vi "StahlPS_Pbus.constructor.vi"(0 "name":string, 2 "data in":string, 5 "error in(no error)":errorcluster) -> (14 "i ref out":refnum<vi>, 16 "data out":string, 19 "error out":errorcluster)   [LabVIEW 2014, in "StahlPS_Pbus.lvlib"]
doc: "This is the constructor of a class.\n\nLicense Agreement for this software:\n\nCopyright (C)\nGesellschaft für Schwerionenforschung, GSI\nPlanckstr. 1\n64291 Darmstadt\nGermany\n\nContact: D.Beck@gsi.de \n\nThis program is free software; you can redistribute it and/or modify it under the terms of the \nGNU General Public License as published by the Free Software Foundation; either version 2 of \nthe license, or (at your option) any later version.\n\nThis program is distributed in the hope that it will be useful, but WITHOUT ANY WARRANTY; \nwithout even the implied warranty of MERCHANTABILITY or FITNESS FOR A PARTICULAR PURPOSE. See the GNU General License for more details (http://www.gnu.org).\n\nGesellschaft für Schwerionenforschung, GSI\nPlanckstr. 1, 64291 Darmstadt, Germany\nFor all questions and ideas contact: M.Richter@gsi.de, H.Brand@gsi.de or D.Beck@gsi.de.\nLast update: 16-JUN-2004"
uses:
  StahlPS_Pbus.lvlib
  CSCore/CSApplicationBaseClasses/DeviceBase/DeviceBase.myEventNames.ctl
  CSCore/CSApplicationBaseClasses/PSChannelBase/PSChannelBase.myEventNames.ctl
  CSlibraries/UtilityLib/UtilityLib.valueStatus.ctl
  CSCore/CSSystem/CSSystemLib/CSSystemLib.lvlib
  CSCore/CSApplicationBaseClasses/PSChannelBase/PSChannelBase.lvlib
  CSCore/CSApplicationBaseClasses/DeviceBase/DeviceBase.lvlib
  CSlibraries/UtilityLib/UtilityLib.lvlib
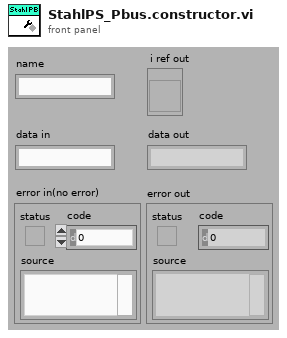
[diagram p1: front panel]
types:
  T1 = typedef "UtilityLib.lvlib/UtilityLib.valueStatus.ctl" = enum16{"no info available", "stand by/off", "on", "warning", "alarm/malfunction", "not implemented", "user action required", "important information", "system default", "control default", "indicator default", "button default"}
  T2 = enum16{"SetAttribute", "GetAttribute", "CreateAttribute", "DestroyAttribute", "DestroyAllAtributes"}
  T3 = typedef "PSChannelBase.lvlib/PSChannelBase.myEventNames.ctl" = enum16{"lvmsg://EmergencyOff", "lvmsg://SetOnOff", "lvmsg://GetOnOff", "lvmsg://SetVoltage", "lvmsg://GetVoltage", "lvmsg://SetCurrent", "lvmsg://GetCurrent", "lvmsg://SetTripCurrent", "lvmsg://GetTripCurrent", "lvmsg://SetRampUpSpeed", "lvmsg://GetRampUpSpeed", "lvmsg://SetRampDownSpeed", "lvmsg://GetRampDownSpeed", "lvmsg://SetChannelOnOff", "lvmsg://GetChannelOnOff", "lvmsg://SetChannelVoltage", "lvmsg://GetChannelVoltage", "lvmsg://SetChannelCurrent", "lvmsg://GetChannelCurrent", "lvmsg://SetChannelTripCurrent", "lvmsg://GetChannelTripCurrent", "lvmsg://SetChannelRampUpSpeed", "lvmsg://GetChannelRampUpSpeed", "lvmsg://SetChannelRampDownSpeed", "lvmsg://GetChannelRampDownSpeed"}
  T4 = typedef "DeviceBase.lvlib/DeviceBase.myEventNames.ctl" = enum16{"lvmsg://Initialize", "lvmsg://Close", "lvmsg://Configure", "lvmsg://Reset", "lvmsg://IDQuery"}
  T5 = typedef "StahlPS_Pbus.lvlib/StahlPS_Pbus.i attribute.ctl" = cluster{"Type":string, "CALC_FACTOR_SET_VOLTAGE":dbl, "CALC_FACTOR_GET_VOLTAGE":dbl, "CALC_FACTOR_GET_CURRENT":dbl, "CALC_FACTOR_SET_CURRENT ":dbl, "REG_VALUE":dbl, "Sign":bool, "setVoltIDs":i32[], "Elektrode Names":string[]}
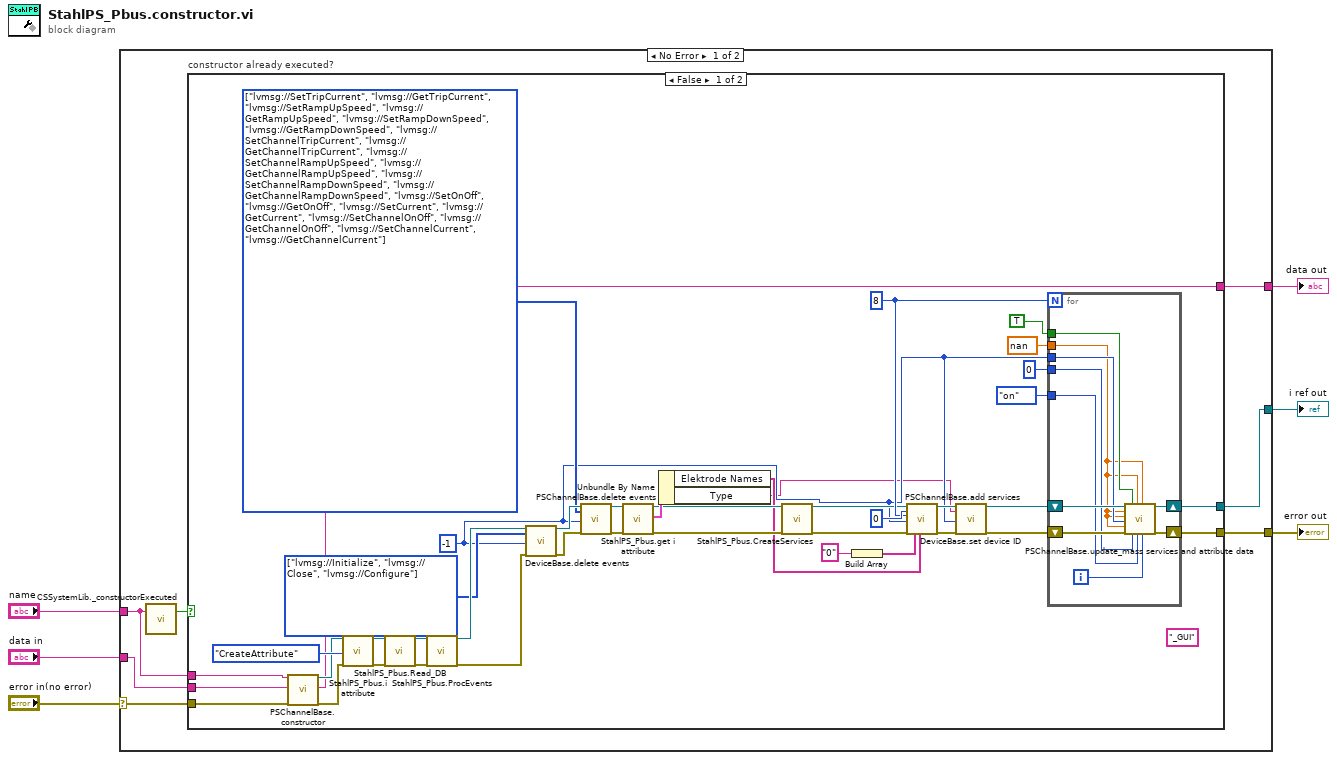
[diagram p0: block diagram]
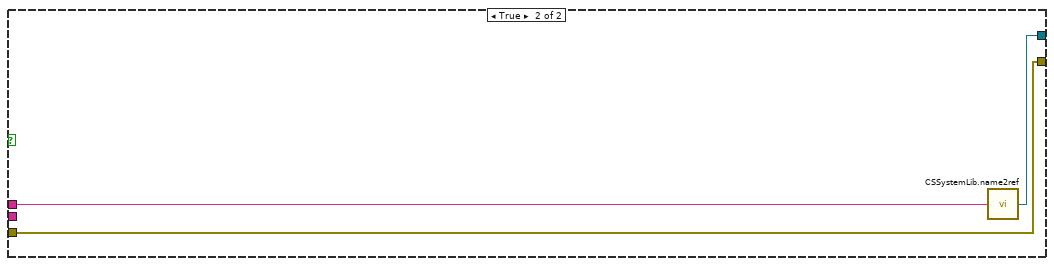
[diagram p2: hidden frame]
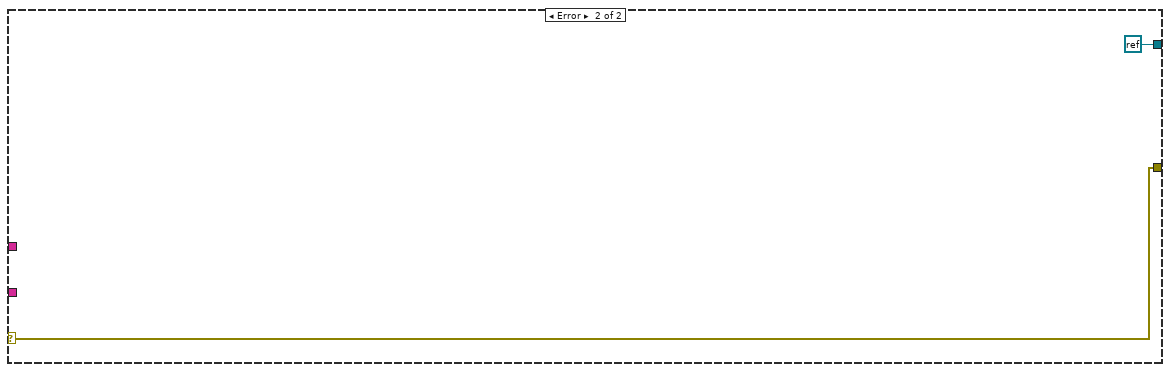
[diagram p3: hidden frame]
diagram:
  n1 = case shown="No Error" "error in(no error)" {
    selector: "error in(no error)" -> [w11 w68]
    tunnel: "name" -> [w10 _]
    tunnel: [w13 refnum<k0> refnum] -> w5
    tunnel: [w12 w68] -> w4
    tunnel: "data in" -> [w8 _]
    tunnel: [w7 _] -> w1
    frame No Error {
      n2 = call "CSSystemLib._constructorExecuted.vi"("name"=w10) -> ("constructor executed?"=w9:bool)  [unwired: 18 in]
      n3 = case "constructor already executed?" shown="False" w9 {
        tunnel: [w31 w66] -> w13
        tunnel: [w32 w65] -> w12
        tunnel: w11 -> [w54 w65]
        tunnel: w10 -> [w19 w67]
        tunnel: w8 -> [w53 _]
        tunnel: [w47 _] -> w7
        frame False {
          (unwired) "_GUI" ("string")
          w39 = T3[] [enum."lvmsg://SetTripCurrent", enum."lvmsg://GetTripCurrent", enum."lvmsg://SetRampUpSpeed", enum."lvmsg://GetRampUpSpeed", enum."lvmsg://SetRampDownSpeed", enum."lvmsg://GetRampDownSpeed", enum."lvmsg://SetChannelTripCurrent", enum."lvmsg://GetChannelTripCurrent", enum."lvmsg://SetChannelRampUpSpeed", enum."lvmsg://GetChannelRampUpSpeed", enum."lvmsg://SetChannelRampDownSpeed", enum."lvmsg://GetChannelRampDownSpeed", enum."lvmsg://SetOnOff", enum."lvmsg://GetOnOff", enum."lvmsg://SetCurrent", enum."lvmsg://GetCurrent", enum."lvmsg://SetChannelOnOff", enum."lvmsg://GetChannelOnOff", enum."lvmsg://SetChannelCurrent", enum."lvmsg://GetChannelCurrent"] items=["lvmsg://EmergencyOff", "lvmsg://SetOnOff", "lvmsg://GetOnOff", "lvmsg://SetVoltage", "lvmsg://GetVoltage", "lvmsg://SetCurrent", "lvmsg://GetCurrent", "lvmsg://SetTripCurrent", "lvmsg://GetTripCurrent", "lvmsg://SetRampUpSpeed", "lvmsg://GetRampUpSpeed", "lvmsg://SetRampDownSpeed", "lvmsg://GetRampDownSpeed", "lvmsg://SetChannelOnOff", "lvmsg://GetChannelOnOff", "lvmsg://SetChannelVoltage", "lvmsg://GetChannelVoltage", "lvmsg://SetChannelCurrent", "lvmsg://GetChannelCurrent", "lvmsg://SetChannelTripCurrent", "lvmsg://GetChannelTripCurrent", "lvmsg://SetChannelRampUpSpeed", "lvmsg://GetChannelRampUpSpeed", "lvmsg://SetChannelRampDownSpeed", "lvmsg://GetChannelRampDownSpeed"] ("events")
          w42 = T4[] [enum."lvmsg://Initialize", enum."lvmsg://Close", enum."lvmsg://Configure"] items=["lvmsg://Initialize", "lvmsg://Close", "lvmsg://Configure", "lvmsg://Reset", "lvmsg://IDQuery"] ("events")
          w27 = 8 ("nofChannels")
          w16 = -1 ("ms timeout (10000)")
          n4 = call "PSChannelBase.constructor.vi"("name"=w19, "data in"=w53, "error in (no error)"=w54) -> ("i ref out"=w48:refnum<vi>, "data out"=w47:string, "error out"=w49:errorcluster)  [unwired: 14 in]
          n5 = call "StahlPS_Pbus.i attribute.vi"("VI Refnum"=w48, "Action"=T2."CreateAttribute", "error in (no error)"=w49) -> ("VI Refnum out"=w51:refnum<vi>, "error out"=w50:errorcluster)  [unwired: 14 in, 1 out]
          n6 = call "StahlPS_Pbus.Read_DB.vi"("i ref in"=w51, "error in (no error)"=w50) -> ("i ref out"=w46:refnum<vi>, "error out (no error)"=w45:errorcluster)  [unwired: 16 in]
          n7 = call "StahlPS_Pbus.ProcEvents.vi"("i ref in"=w46, "error in"=w45) -> ("i ref out"=w44:refnum<vi>, "error out"=w43:errorcluster)  [unwired: 16 in]
          n8 = call "DeviceBase.delete events.vi"("i ref in"=w44, "events"=w42, "ms timeout (10000)"=w16, "error in (no error)"=w43) -> ("i ref out"=w41:refnum<vi>, "error out"=w40:errorcluster)  [unwired: 13 in, 1 out]
          n9 = call "PSChannelBase.delete events.vi"("i ref in"=w41, "events"=w39, "ms timeout (10000)"=w16, "error in (no error)"=w40) -> ("i ref out"=w36:refnum<vi>, "error out"=w37:errorcluster)  [unwired: 13 in, 1 out]
          n10 = call "StahlPS_Pbus.get i attribute.vi"("i ref in"=w36, "error in (no error)"=w37) -> ("i ref out"=w17:refnum<vi>, "i attribute"=w35:T5, "error out"=w18:errorcluster)  [unwired: 15 in]
          n11 = Unbundle By Name(w35) -> ("Elektrode Names"=w15:string[], "Type"=w14:string)
          n12 = call "StahlPS_Pbus.CreateServices.vi"("i ref in"=w17, "error in(no error)"=w18) -> ("i ref out"=w21:refnum<vi>, "error out"=w22:errorcluster)  [unwired: 16 in]
          n13 = Build Array("0") -> (w33:string[])
          n14 = call "PSChannelBase.add services.vi"("i ref in"=w21, "defaultChannelIndex"=0, "nofChannels"=w27, "ms timeout (10000)"=w16, "error in (no error)"=w22, "physicalNames"=w33, "logicalNames"=w15) -> ("i ref out"=w26:refnum<vi>, "error out"=w24:errorcluster)  [unwired: 10 in, 1 out]
          n15 = call "DeviceBase.set device ID.vi"("i ref in"=w26, "deviceID"=w14, "ms timeout (10000)"=w16, "error in (no error)"=w24) -> ("i ref out"=w25:refnum<vi>, "error out"=w23:errorcluster)  [unwired: 13 in, 1 out]
          n16 = for {
            N: w27 -> [_]
            shift-right: [w62] -> w32
            shift-left: w23 -> [w63]
            shift-right: [w60] -> w31
            shift-left: w25 -> [w61]
            tunnel: UtilityLib.valueStatus."on" ("valueStatus") -> [w59]
            tunnel: nan -> [w56]
            tunnel: w16 -> [w58]
            tunnel: TRUE -> [w57]
            tunnel: 0 -> [w55]
            i -> [w64]
            n17 = call "PSChannelBase.update_mass services and attribute data.vi"("i ref in"=w61, "tripCurrent"=w56, "rampUpSpeed"=w56, "ms timeout (10000)"=w58, "rampDownSpeed"=w56, "error in (no error)"=w63, "onOff"=w57, "status"=w55, "voltage"=w56, "valueStatus"=w59, "current"=w56, "channelNumber"=w64) -> ("i ref out"=w60:refnum<vi>, "error out"=w62:errorcluster)  [unwired: 5 in, 1 out]
          }
        }
        frame True {
          n18 = call "CSSystemLib.name2ref.vi"("name"=w67) -> ("obj refnum"=w66:refnum<vi>)
        }
      }
    }
    frame Error {
    }
  }
  "i ref out" <- w5
  "error out" <- w4
  "data out" <- w1
